vi "Target Fnc & Deriv NonLin.vi"(2 "X":dbl format="%0.3f", 3 "Coefficients":dbl[](array[numeric]) format="%0.5f", 4 "Flag":enum16{"no deriv", "deriv"}(ring)) -> (0 "Derivatives":dbl[](array[numeric]) format="%0.5f", 1 "Y":dbl format="%0.3f")   [LabVIEW 2020, in "NI_AALPro.lvlib"]
doc: "Here the user specifies his guess at the functional form of the relationship between Y and X as a function of coefficients. \n\nIf the partial derivatives of the function are known, the user also furnishes the equations for the partial derivatives of this function with respect to each coefficient. The input control Flag should then be set to 1 (deriv) by all calling VIs.\n\nIf the partial derivatives of the function are not known, the input control Flag should be set to 0 (no deriv) by all calling VIs, and a numerical approximation to the partial derivatives will be computed."
uses:
  <vilib>/Analysis/NI_AALPro.lvlib
panel:
  # "This VI calculates the output Y as a function of the input array X as well as the derivatives of the function at all values of X. The user specifies the \"Target Function\" and its derivatives in the formula nodes of this VI. The function describes the relationship of Y to X and the coefficients used are updated in each iteration after a new guess at their value is taken. Hence Y, Derivatives, and Coefficients are continuously changing."
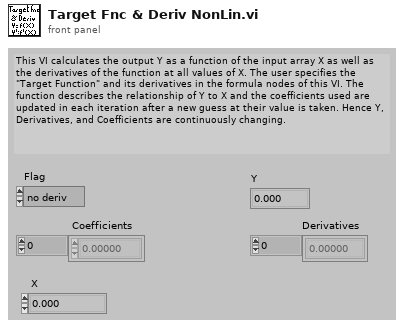
[diagram p1: front panel]
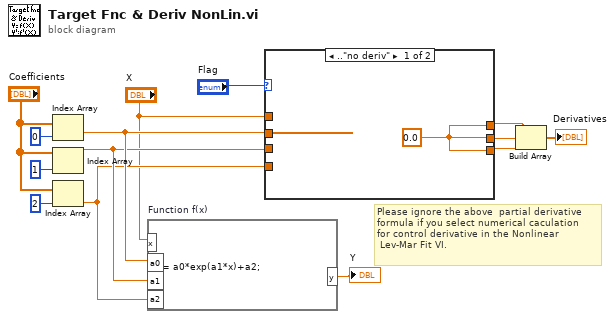
[diagram p0: block diagram]
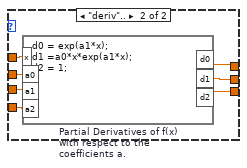
[diagram p2: hidden frame]
diagram:
  # "Please ignore the above  partial derivative \nformula if you select numerical caculation \nfor control derivative in the Nonlinear\n Lev-Mar Fit VI."
  n1 = Index Array(array="Coefficients", index=0) -> (element=w10:dbl)
  n2 = Index Array(array="Coefficients", index=1) -> (element=w9:dbl)
  n3 = Index Array(array="Coefficients", index=2) -> (element=w8:dbl)
  n4 = formula code="y= a0*exp(a1*x)+a2;" "Function f(x)"("x"="X", "a0"=w10, "a1"=w9, "a2"=w8) -> ("y"=→"Y":dbl)
  n5 = case shown="..\"no deriv\"" "Flag" {
    tunnel: "X" -> [_ w16]
    tunnel: [w15 w17] -> w5
    tunnel: [w15 w18] -> w6
    tunnel: [w15 w19] -> w7
    tunnel: w8 -> [_ w20]
    tunnel: w9 -> [_ w21]
    tunnel: w10 -> [_ w22]
    frame .."no deriv" {
      w15 = 0.0
    }
    frame "deriv".. {
      n6 = formula code="d0 = exp(a1*x);\nd1 =a0*x*exp(a1*x);\nd2 = 1;" "Partial Derivatives of f(x) with respect to the coefficients a."("x"=w16, "a0"=w22, "a1"=w21, "a2"=w20) -> ("d0"=w19:dbl, "d1"=w18:dbl, "d2"=w17:dbl)
    }
  }
  n7 = Build Array(w7, w6, w5) -> (→"Derivatives":dbl[])
